vi "X Axis Motor state control subVI.vi"(8 "error in (no error)":errorcluster, 10 "stop":bool, 11 "X Axis Motor Target":T1) -> (0 "error out":errorcluster, 3 "X Axis Motor Params":T2)   [LabVIEW 2018]
uses:
  Motor Status Enum.ctl
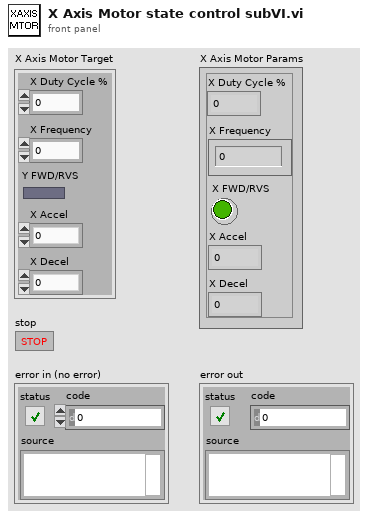
[diagram p1: front panel]
types:
  T1 = cluster{"X Frequency":dbl, "Y FWD/RVS":bool, "X Accel":dbl, "X Decel":dbl, "X Duty Cycle %":dbl}
  T2 = cluster{"X Frequency":dbl, "X FWD/RVS":bool, "X Accel":dbl, "X Decel":dbl, "X Duty Cycle %":dbl}
  T3 = cluster{"X Frequency":dbl, "X FWD/RVS":bool, "Accel":dbl, "Decel":dbl, "X Duty %":dbl}
  T4 = typedef "Motor Status Enum.ctl" = enum16{"Stop Motor", "Read Inputs", "Steady Speed", "Accelerate", "Decelerate"}
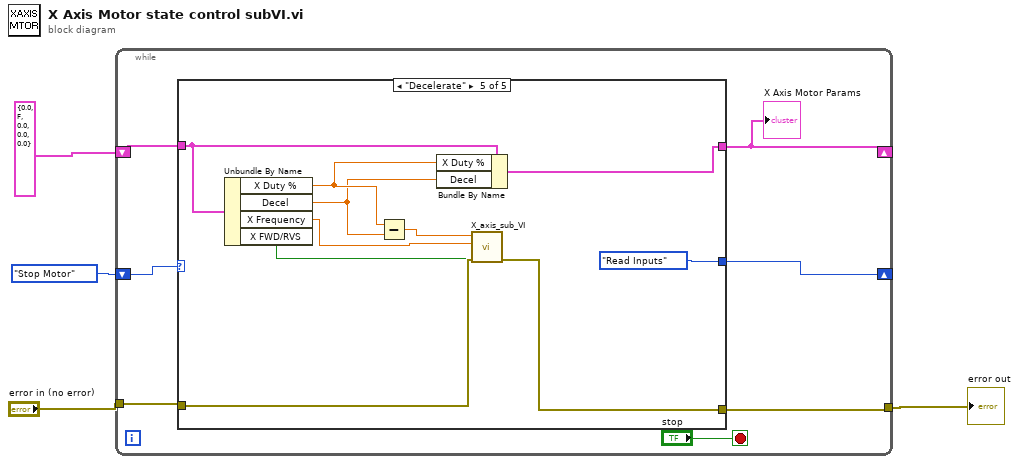
[diagram p0: block diagram]
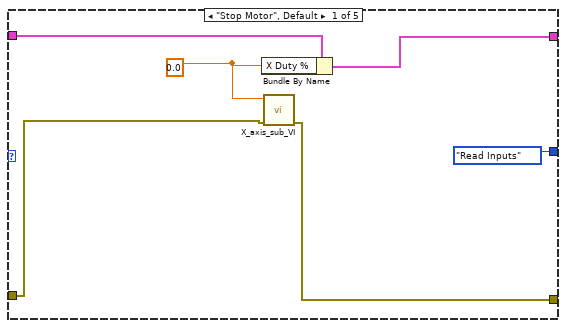
[diagram p2: hidden frame]
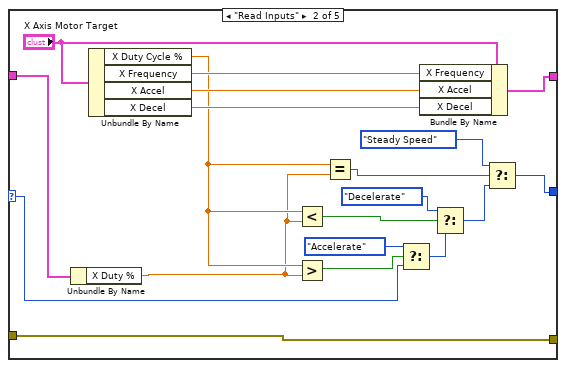
[diagram p3: hidden frame]
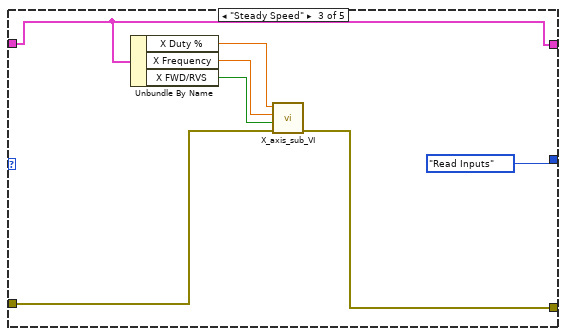
[diagram p4: hidden frame]
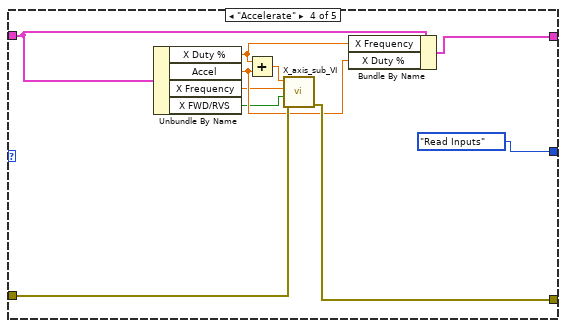
[diagram p5: hidden frame]
diagram:
  n1 = while {
    shift-right: [w5] -> _
    shift-left: T3 {"X Frequency"=0.0, "X FWD/RVS"=FALSE, "Accel"=0.0, "Decel"=0.0, "X Duty %"=0.0} ("X Axis Motor Params 2") -> [w6]
    tunnel: "error in (no error)" -> [w9]
    tunnel: [w8] -> w3
    shift-right: [w7] -> _
    shift-left: Motor_Status_Enum."Stop Motor" -> [w10]
    stop <- "stop" stop-if-true
    n2 = case shown="\"Decelerate\"" w10 {
      selector: w10 -> [_ w18 _ _ _]
      tunnel: w9 -> [w14 w36 w39 w53 w58]
      tunnel: [w12 w36 w38 w52 w57] -> w8
      tunnel: [Motor_Status_Enum."Read Inputs" w23 Motor_Status_Enum."Read Inputs" Motor_Status_Enum."Read Inputs" Motor_Status_Enum."Read Inputs"] -> w7
      tunnel: w6 -> [w16 w30 w41 w49 w60]
      tunnel: [w15 w35 w41 w48 w59] -> w5
      frame "Stop Motor", Default {
        w13 = 0.0 ("Y Frequency")
        n3 = Bundle By Name(cluster=w16, "X Duty %"=w13) -> (w15:T3)
        n4 = call "X_axis_sub_VI.vi"("error in (no error)"=w14, "Duty Cycle %"=w13) -> ("error out"=w12:errorcluster)  [unwired: 9 in]
      }
      frame "Read Inputs" {
        n5 = Unbundle By Name(w30) -> ("X Duty %"=w20:dbl)
        n6 = Unbundle By Name("X Axis Motor Target") -> ("X Duty Cycle %"=w21:dbl, "X Frequency"=w31:dbl, "X Accel"=w33:dbl, "X Decel"=w32:dbl)
        n7 = Less?(x=w21, y=w20) -> (x < y?=w27:bool)
        n8 = Greater?(x=w21, y=w20) -> (0:w29:bool)
        n9 = Equal?(x=w21, y=w20) -> (x = y?=w22:bool)
        n10 = Select(t=Motor_Status_Enum."Accelerate", s=w29, f=w18) -> (s? t:f=w25:T4)
        n11 = Bundle By Name(cluster="X Axis Motor Target", "X Frequency"=w31, "X Accel"=w33, "X Decel"=w32) -> (w35:T1)
        n12 = Select(t=Motor_Status_Enum."Decelerate", s=w27, f=w25) -> (s? t:f=w24:T4)
        n13 = Select(t=Motor_Status_Enum."Steady Speed", s=w22, f=w24) -> (s? t:f=w23:T4)
      }
      frame "Steady Speed" {
        n14 = Unbundle By Name(w41) -> ("X Duty %"=w37:dbl, "X Frequency"=w43:dbl, "X FWD/RVS"=w42:bool)
        n15 = call "X_axis_sub_VI.vi"("error in (no error)"=w39, "FWD/RVS"=w42, "Frequency"=w43, "Duty Cycle %"=w37) -> ("error out"=w38:errorcluster)  [unwired: 7 in]
      }
      frame "Accelerate" {
        n16 = Unbundle By Name(w49) -> ("X Duty %"=w47:dbl, "Accel"=w46:dbl, "X Frequency"=w45:dbl, "X FWD/RVS"=w44:bool)
        n17 = Add(x=w47, y=w46) -> (x+y=w50:dbl)
        n18 = call "X_axis_sub_VI.vi"("error in (no error)"=w53, "FWD/RVS"=w44, "Frequency"=w45, "Duty Cycle %"=w50) -> ("error out"=w52:errorcluster)  [unwired: 7 in]
        n19 = Bundle By Name(cluster=w49, "X Frequency"=w47, "X Duty %"=w46) -> (w48:T3)
      }
      frame "Decelerate" {
        n20 = Unbundle By Name(w60) -> ("X Duty %"=w62:dbl, "Decel"=w61:dbl, "X Frequency"=w55:dbl, "X FWD/RVS"=w54:bool)
        n21 = Subtract(x=w62, y=w61) -> (x-y=w63:dbl)
        n22 = Bundle By Name(cluster=w60, "X Duty %"=w62, "Decel"=w61) -> (w59:T3)
        n23 = call "X_axis_sub_VI.vi"("error in (no error)"=w58, "FWD/RVS"=w54, "Frequency"=w55, "Duty Cycle %"=w63) -> ("error out"=w57:errorcluster)  [unwired: 7 in]
      }
    }
    "X Axis Motor Params" <- w5
  }
  "error out" <- w3
